vi "6-11-19 Decreasing Temp.vi"() -> ()   [LabVIEW 2016]
uses:
  <vilib>/Analysis/baseanly.llb/Mean (DBL).vi
  <userlib>/Levylab/LV to ITX/LVtoITX.lvclass
  <vilib>/Analysis/NI_AALPro.lvlib
  <vilib>/Analysis/NI_AALBase.lvlib
panel:
  out "M4T":dbl[](array[numeric])
  out "M2T":dbl[](array[numeric])
  out "M/G v Temp":T1(graph)
  out "M/G vs Temp Normalized vs 275":cluster{dbl[], dbl[]}[](graph)
  out "M/G vs Temp Normalized vs prev":cluster{dbl[], dbl[]}[](graph)
  in  "parameter bounds":T2={"slope min"=-inf, "slope max"=inf, "intercept min"=-inf, "intercept max"=inf}
  out "Fits":T1(graph)
  out "Temp vs Time":cluster{"Data":dbl[], "Data":dbl[]}(graph)
  out "G vs Temp":cluster{"Data":dbl[], "Data":dbl[]}[](graph)
  in  "Path":path=path "G:/My Drive/Data/6-11 Decreasing SA40060.dat"
  out "Wavenames":string[](array[string])
  out "Comments":string
  in  "header length":i32=37
  out "G vs Time":cluster{"Data":dbl[], "Data":dbl[]}[](graph)
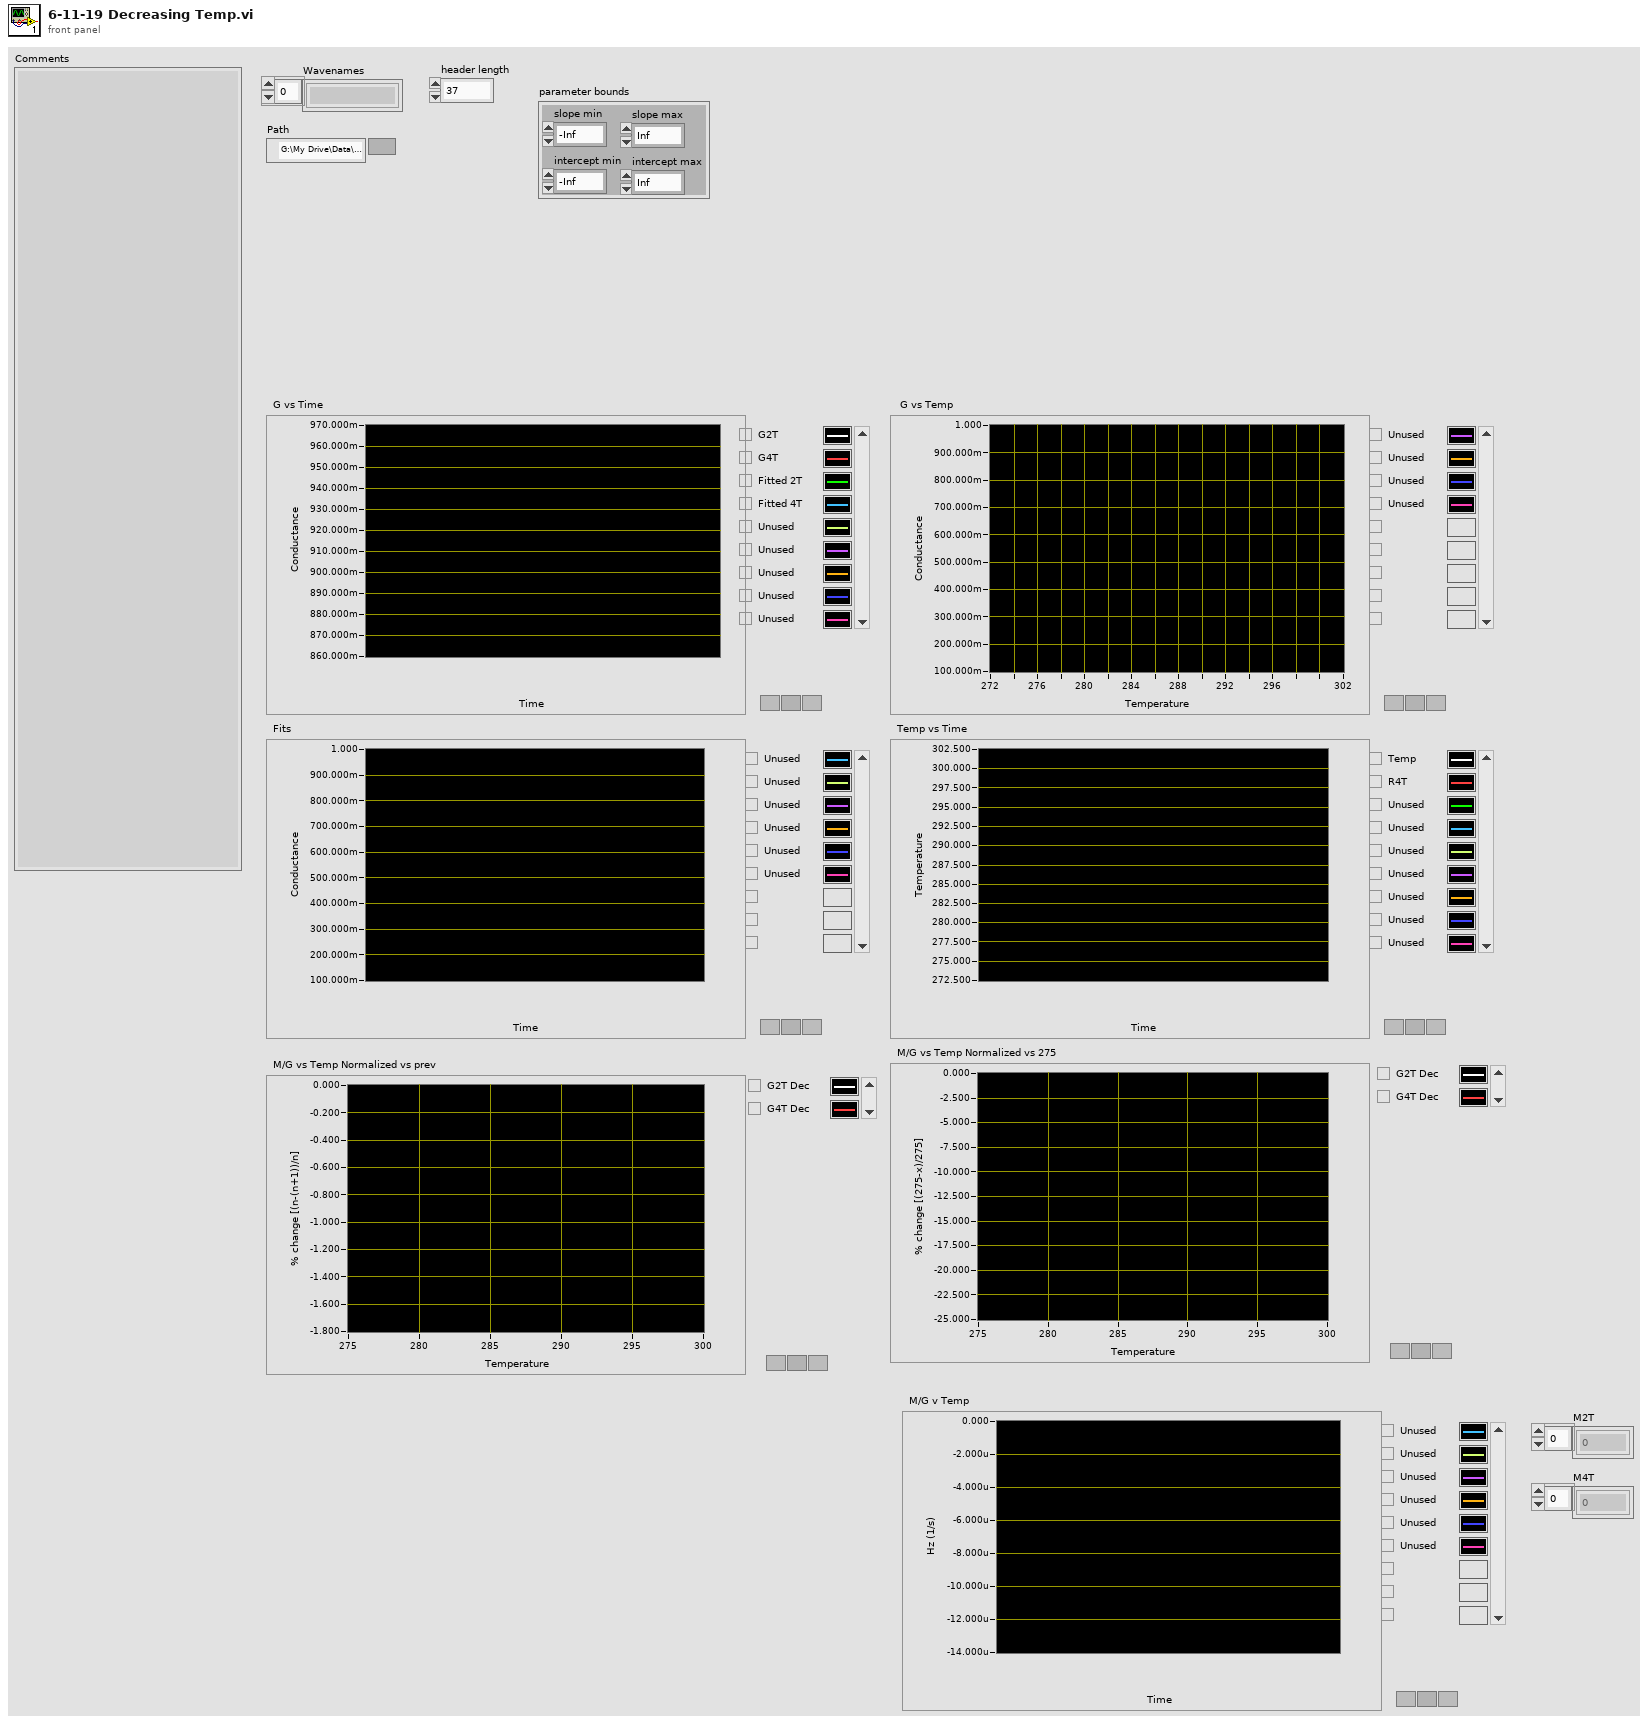
[diagram p1: front panel]
types:
  T1 = cluster{"Data":dbl[], "Best Exponential Fit":dbl[]}[]
  T2 = cluster{"slope min":dbl, "slope max":dbl, "intercept min":dbl, "intercept max":dbl}
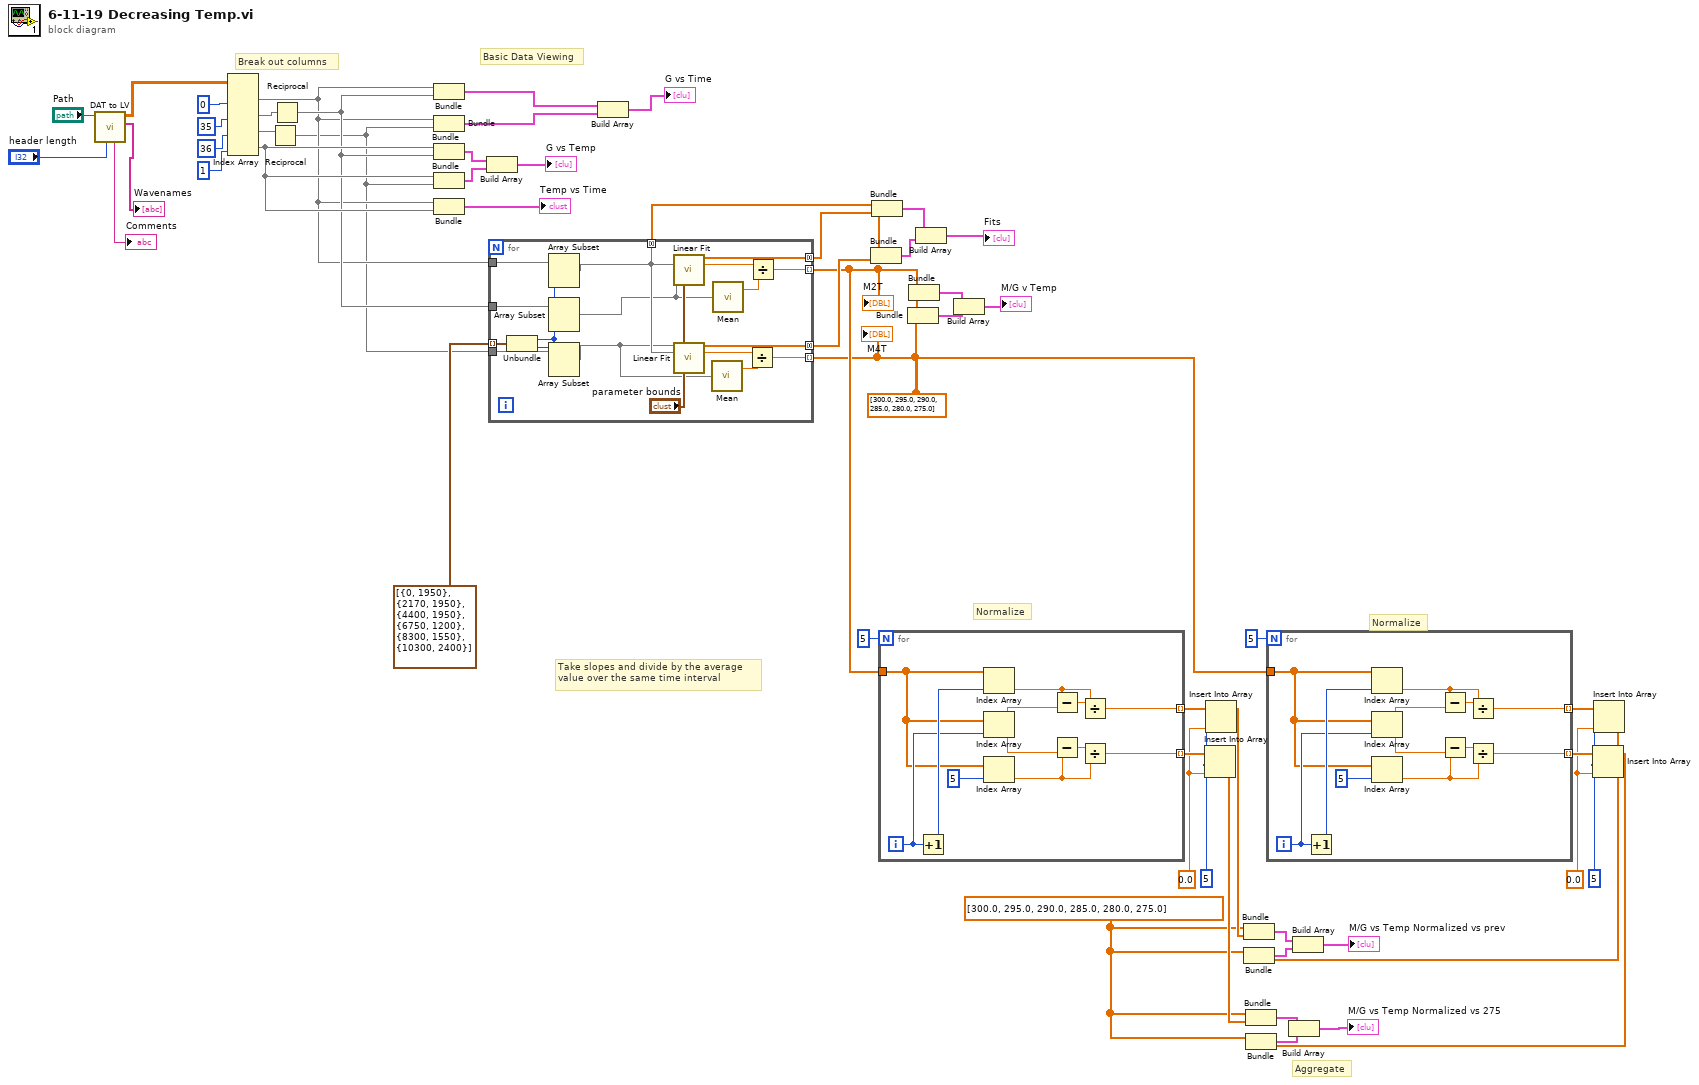
[diagram p0: block diagram]
diagram:
  w2 = dbl[] [300.0, 295.0, 290.0, 285.0, 280.0, 275.0]
  w10 = 5
  w11 = 0.0
  w19 = 5
  w20 = 0.0
  w7 = dbl[] [300.0, 295.0, 290.0, 285.0, 280.0, 275.0]
  # "Aggregate"
  # "Normalize"
  # "Normalize"
  # "Take slopes and divide by the average \nvalue over the same time interval"
  # "Basic Data Viewing"
  # "Break out columns"
  n1 = call <userlib>:"DAT to LV.vi"("header length"="header length", "File Path"="Path") -> ("Wavenames"=→"Wavenames":string[], "Data"=w48:dbl[][], "Comments"=→"Comments":string)  [unwired: 6 in, 1 out]
  n2 = Index Array(array=w48, index (col) #1=0 ("disabled index (col)"), index (col) #2=35 ("index (col)"), index (col) #3=36 ("index (col)"), index (col) #4=1 ("index (col)")) -> (element #1=w28:dbl[], element #2=w39:dbl[], element #3=w40:dbl[], element #4=w30:dbl[])  [unwired: 4 in]
  n3 = Reciprocal(x=w40) -> (1/x=w27:dbl[])
  n4 = Reciprocal(x=w39) -> (1/x=w29:dbl[])
  n5 = Bundle("Data"=w28, w29) -> (w47:cluster{"Data":dbl[], dbl[]})  [unwired: 1 in]
  n6 = Bundle("Data"=w28, w27) -> (w46:cluster{"Data":dbl[], dbl[]})  [unwired: 1 in]
  n7 = Bundle("Data"=w30, w29) -> (w44:cluster{"Data":dbl[], dbl[]})  [unwired: 1 in]
  n8 = Bundle("Data"=w30, w27) -> (w45:cluster{"Data":dbl[], dbl[]})  [unwired: 1 in]
  n9 = Bundle("Data"=w28, "Data"=w30) -> (→"Temp vs Time":cluster{"Data":dbl[], "Data":dbl[]})  [unwired: 1 in]
  n10 = Build Array(w44, w45) -> (→"G vs Temp":cluster{"Data":dbl[], dbl[]}[])
  n11 = for {
    tunnel: cluster{"index":i32, "length":i32}[] [{"index"=0, "length"=1950}, {"index"=2170, "length"=1950}, {"index"=4400, "length"=1950}, {"index"=6750, "length"=1200}, {"index"=8300, "length"=1550}, {"index"=10300, "length"=2400}] -> [w74] mode=indexing
    tunnel: [w60] -> w4 mode=indexing
    tunnel: [w59] -> w3 mode=indexing
    tunnel: [w73] -> w33 mode=concatenating
    tunnel: [w72] -> w41 mode=concatenating
    tunnel: w29 -> [w70]
    tunnel: w27 -> [w69]
    tunnel: w28 -> [w68]
    tunnel: [w66] -> w15 mode=concatenating
    n12 = Unbundle(w74) -> ("index"=w67:i32, "length"=w71:i32)
    n13 = Array Subset(array=w68, index=w67, length=w71) -> (w66:dbl[])
    n14 = Array Subset(array=w70, index=w67, length=w71) -> (w64:dbl[])
    n15 = Array Subset(array=w69, index=w67, length=w71) -> (w63:dbl[])
    n16 = call <vilib>:"Linear Fit.vi"("Y"=w64, "X"=w66, "parameter bounds"="parameter bounds") -> ("Best Linear Fit"=w72:dbl[], "slope"=w62:dbl)  [unwired: 8 in, 3 out]
    n17 = call <vilib>:"Linear Fit.vi"("Y"=w63, "X"=w66, "parameter bounds"="parameter bounds") -> ("Best Linear Fit"=w73:dbl[], "slope"=w58:dbl)  [unwired: 8 in, 3 out]
    n18 = call-poly <vilib>:"Mean.vi"("X"=w63) -> ("mean"=w57:dbl)  [unwired: 1 out]
    n19 = call-poly <vilib>:"Mean.vi"("X"=w64) -> ("mean"=w61:dbl)  [unwired: 1 out]
    n20 = Divide(x=w58, y=w57) -> (x/y=w59:dbl)
    n21 = Divide(x=w62, y=w61) -> (x/y=w60:dbl)
  }
  "M2T" <- w4
  "M4T" <- w3
  n22 = Build Array(w47, w46) -> (→"G vs Time":cluster{"Data":dbl[], dbl[]}[])
  n23 = Bundle(w15, "Best Linear Fit"=w33) -> (w37:cluster{dbl[], "Best Linear Fit":dbl[]})  [unwired: 1 in]
  n24 = Bundle(w15, "Best Linear Fit"=w41) -> (w38:cluster{dbl[], "Best Linear Fit":dbl[]})  [unwired: 1 in]
  n25 = for {
    N: 5 -> [_]
    tunnel: w4 -> [w82]
    tunnel: [w79] -> w22 mode=indexing
    tunnel: [w78] -> w21 mode=indexing
    i -> [w84]
    n26 = Increment(x=w84) -> (x+1=w85:i32)
    n27 = Index Array(array=w82, index=w85) -> (element=w77:dbl)
    n28 = Index Array(array=w82, index=w84) -> (element=w76:dbl)
    n29 = Index Array(array=w82, index=5) -> (element=w75:dbl)
    n30 = Subtract(x=w77, y=w76) -> (x-y=w81:dbl)
    n31 = Subtract(x=w75, y=w76) -> (x-y=w80:dbl)
    n32 = Divide(x=w81, y=w77) -> (x/y=w78:dbl)
    n33 = Divide(x=w80, y=w75) -> (x/y=w79:dbl)
  }
  n34 = Bundle(w2, w3) -> (w6:cluster{dbl[], dbl[]})  [unwired: 1 in]
  n35 = Bundle(w2, w4) -> (w5:cluster{dbl[], dbl[]})  [unwired: 1 in]
  n36 = Build Array(w38, w37) -> (→"Fits":cluster{dbl[], "Best Linear Fit":dbl[]}[])
  n37 = Build Array(w5, w6) -> (→"M/G v Temp":cluster{dbl[], dbl[]}[])
  n38 = Insert Into Array(array=w22, index=w19, new element=w20) -> (w16:dbl[])
  n39 = Insert Into Array(array=w21, index=w19, new element=w20) -> (w14:dbl[])
  n40 = Bundle(w7, w14) -> (w32:cluster{dbl[], dbl[]})  [unwired: 1 in]
  n41 = Bundle(w7, w16) -> (w26:cluster{dbl[], dbl[]})  [unwired: 1 in]
  n42 = for {
    N: 5 -> [_]
    tunnel: w3 -> [w93]
    tunnel: [w90] -> w12 mode=indexing
    tunnel: [w89] -> w13 mode=indexing
    i -> [w95]
    n43 = Increment(x=w95) -> (x+1=w96:i32)
    n44 = Index Array(array=w93, index=w96) -> (element=w87:dbl)
    n45 = Index Array(array=w93, index=w95) -> (element=w86:dbl)
    n46 = Index Array(array=w93, index=5) -> (element=w88:dbl)
    n47 = Subtract(x=w87, y=w86) -> (x-y=w92:dbl)
    n48 = Subtract(x=w88, y=w86) -> (x-y=w91:dbl)
    n49 = Divide(x=w92, y=w87) -> (x/y=w89:dbl)
    n50 = Divide(x=w91, y=w88) -> (x/y=w90:dbl)
  }
  n51 = Insert Into Array(array=w12, index=w10, new element=w11) -> (w8:dbl[])
  n52 = Bundle(w7, w8) -> (w25:cluster{dbl[], dbl[]})  [unwired: 1 in]
  n53 = Build Array(w26, w25) -> (→"M/G vs Temp Normalized vs 275":cluster{dbl[], dbl[]}[])
  n54 = Insert Into Array(array=w13, index=w10, new element=w11) -> (w9:dbl[])
  n55 = Bundle(w7, w9) -> (w31:cluster{dbl[], dbl[]})  [unwired: 1 in]
  n56 = Build Array(w32, w31) -> (→"M/G vs Temp Normalized vs prev":cluster{dbl[], dbl[]}[])
